vi "HARDWARE.vi"(8 "error in (no error)":errorcluster, 10 "Caracter Servicio":string="b", 11 "Turnos in":refnum<class "Turnos.lvclass">) -> (0 "error out":errorcluster, 3 "Turnos out":refnum<class "Turnos.lvclass">)   [LabVIEW 2020, in "Turnos.lvlib" / "Turnos.lvclass"]
uses:
  Turnos.lvclass
  <vilib>/Instr/_visa.llb/VISA Configure Serial Port (Instr).vi
  Turnos.lvclass/Turnos.ctl
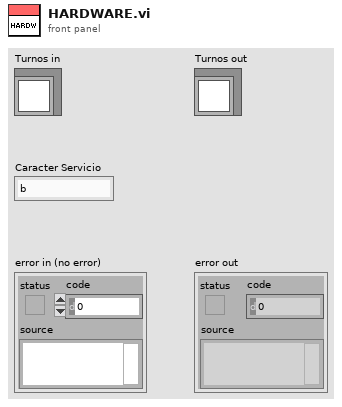
[diagram p1: front panel]
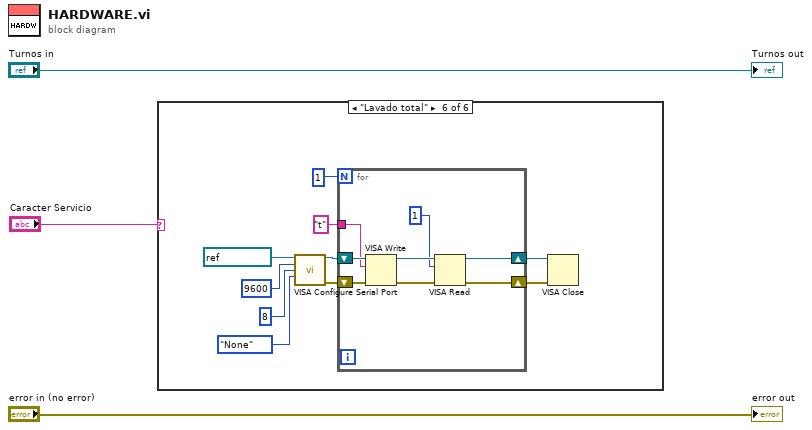
[diagram p0: block diagram]
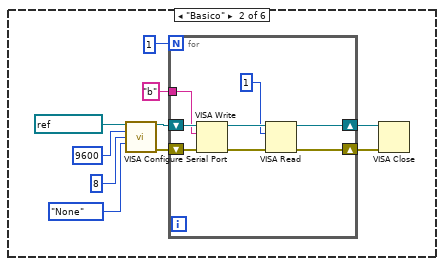
[diagram p3: hidden frame]
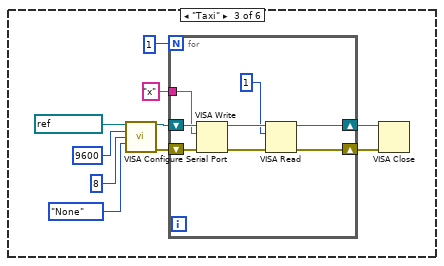
[diagram p4: hidden frame]
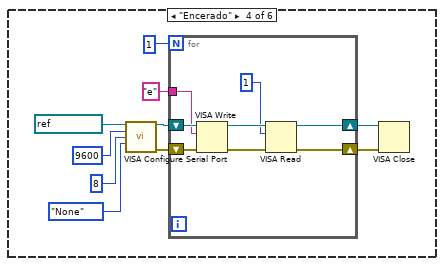
[diagram p5: hidden frame]
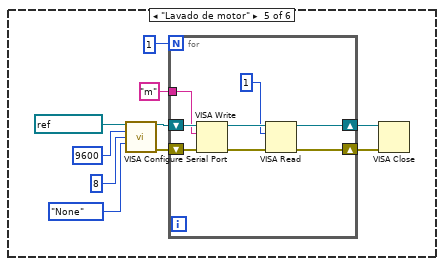
[diagram p6: hidden frame]
diagram:
  n1 = case shown="\"Lavado total\"" "Caracter Servicio" {
    frame "False", Default {
    }
    frame "Basico" {
      n2 = call-poly "VISA Configure Serial Port"("VISA resource name"=refnum<visa-resource-name> "COM10" ("Serial"), "baud rate (9600)"=u32 9600, "data bits (8)"=u16 8, "parity (0:none)"=enum16{"None", "Odd", "Even", "Mark", "Space"}."None") -> ("VISA resource name out"=w7:refnum<visa-resource-name>, "error out"=w6:errorcluster)  [unwired: 10 in]
      n3 = for {
        N: 1 -> [_]
        shift-right: [w21] -> w13
        shift-left: w7 -> [w19]
        shift-right: [w20] -> w12
        shift-left: w6 -> [w18]
        tunnel: "b" ("Caracter Servicio") -> [w14]
        n4 = VISA Write(VISA resource name=w19, write buffer=w14, error in (no error)=w18) -> (VISA resource name out=w17:refnum<visa-resource-name>, error out=w16:errorcluster)  [unwired: 1 out]
        n5 = VISA Read(VISA resource name=w17, byte count=u32 1, error in (no error)=w16) -> (VISA resource name out=w21:refnum<visa-resource-name>, error out=w20:errorcluster)  [unwired: 2 out]
      }
      n6 = VISA Close(VISA resource name=w13, error in (no error)=w12) -> ()  [unwired: 1 out]
    }
    frame "Taxi" {
      n7 = call-poly "VISA Configure Serial Port"("VISA resource name"=refnum<visa-resource-name> "COM10" ("Serial"), "baud rate (9600)"=u32 9600, "data bits (8)"=u16 8, "parity (0:none)"=enum16{"None", "Odd", "Even", "Mark", "Space"}."None") -> ("VISA resource name out"=w25:refnum<visa-resource-name>, "error out"=w24:errorcluster)  [unwired: 10 in]
      n8 = for {
        N: 1 -> [_]
        shift-right: [w39] -> w31
        shift-left: w25 -> [w37]
        shift-right: [w38] -> w30
        shift-left: w24 -> [w36]
        tunnel: "x" ("Caracter Servicio") -> [w32]
        n9 = VISA Write(VISA resource name=w37, write buffer=w32, error in (no error)=w36) -> (VISA resource name out=w35:refnum<visa-resource-name>, error out=w34:errorcluster)  [unwired: 1 out]
        n10 = VISA Read(VISA resource name=w35, byte count=u32 1, error in (no error)=w34) -> (VISA resource name out=w39:refnum<visa-resource-name>, error out=w38:errorcluster)  [unwired: 2 out]
      }
      n11 = VISA Close(VISA resource name=w31, error in (no error)=w30) -> ()  [unwired: 1 out]
    }
    frame "Encerado" {
      n12 = call-poly "VISA Configure Serial Port"("VISA resource name"=refnum<visa-resource-name> "COM10" ("Serial"), "baud rate (9600)"=u32 9600, "data bits (8)"=u16 8, "parity (0:none)"=enum16{"None", "Odd", "Even", "Mark", "Space"}."None") -> ("VISA resource name out"=w43:refnum<visa-resource-name>, "error out"=w42:errorcluster)  [unwired: 10 in]
      n13 = for {
        N: 1 -> [_]
        shift-right: [w57] -> w49
        shift-left: w43 -> [w55]
        shift-right: [w56] -> w48
        shift-left: w42 -> [w54]
        tunnel: "e" ("Caracter Servicio") -> [w50]
        n14 = VISA Write(VISA resource name=w55, write buffer=w50, error in (no error)=w54) -> (VISA resource name out=w53:refnum<visa-resource-name>, error out=w52:errorcluster)  [unwired: 1 out]
        n15 = VISA Read(VISA resource name=w53, byte count=u32 1, error in (no error)=w52) -> (VISA resource name out=w57:refnum<visa-resource-name>, error out=w56:errorcluster)  [unwired: 2 out]
      }
      n16 = VISA Close(VISA resource name=w49, error in (no error)=w48) -> ()  [unwired: 1 out]
    }
    frame "Lavado de motor" {
      n17 = call-poly "VISA Configure Serial Port"("VISA resource name"=refnum<visa-resource-name> "COM10" ("Serial"), "baud rate (9600)"=u32 9600, "data bits (8)"=u16 8, "parity (0:none)"=enum16{"None", "Odd", "Even", "Mark", "Space"}."None") -> ("VISA resource name out"=w61:refnum<visa-resource-name>, "error out"=w60:errorcluster)  [unwired: 10 in]
      n18 = for {
        N: 1 -> [_]
        shift-right: [w75] -> w67
        shift-left: w61 -> [w73]
        shift-right: [w74] -> w66
        shift-left: w60 -> [w72]
        tunnel: "m" ("Caracter Servicio") -> [w68]
        n19 = VISA Write(VISA resource name=w73, write buffer=w68, error in (no error)=w72) -> (VISA resource name out=w71:refnum<visa-resource-name>, error out=w70:errorcluster)  [unwired: 1 out]
        n20 = VISA Read(VISA resource name=w71, byte count=u32 1, error in (no error)=w70) -> (VISA resource name out=w75:refnum<visa-resource-name>, error out=w74:errorcluster)  [unwired: 2 out]
      }
      n21 = VISA Close(VISA resource name=w67, error in (no error)=w66) -> ()  [unwired: 1 out]
    }
    frame "Lavado total" {
      n22 = call-poly "VISA Configure Serial Port"("VISA resource name"=refnum<visa-resource-name> "COM10" ("Serial"), "baud rate (9600)"=u32 9600, "data bits (8)"=u16 8, "parity (0:none)"=enum16{"None", "Odd", "Even", "Mark", "Space"}."None") -> ("VISA resource name out"=w79:refnum<visa-resource-name>, "error out"=w78:errorcluster)  [unwired: 10 in]
      n23 = for {
        N: 1 -> [_]
        shift-right: [w93] -> w85
        shift-left: w79 -> [w91]
        shift-right: [w92] -> w84
        shift-left: w78 -> [w90]
        tunnel: "t" ("Caracter Servicio") -> [w86]
        n24 = VISA Write(VISA resource name=w91, write buffer=w86, error in (no error)=w90) -> (VISA resource name out=w89:refnum<visa-resource-name>, error out=w88:errorcluster)  [unwired: 1 out]
        n25 = VISA Read(VISA resource name=w89, byte count=u32 1, error in (no error)=w88) -> (VISA resource name out=w93:refnum<visa-resource-name>, error out=w92:errorcluster)  [unwired: 2 out]
      }
      n26 = VISA Close(VISA resource name=w85, error in (no error)=w84) -> ()  [unwired: 1 out]
    }
  }
  "error out" <- "error in (no error)"
  "Turnos out" <- "Turnos in"
